vi "Generate Signature.vi"(8 "error in (no error)":errorcluster, 9 "Key":string, 10 "Message":string, 11 "HMAC in":refnum<class "HMAC.lvclass">) -> (0 "error out":errorcluster, 2 "Signature":string, 3 "HMAC out":refnum<class "HMAC.lvclass">)   [LabVIEW 2018, in "Crypto.lvlib" / "HMAC.lvclass"]
uses:
  HMAC.lvclass
  HMAC.lvclass/HMAC.ctl
  Hash/Hash.lvclass
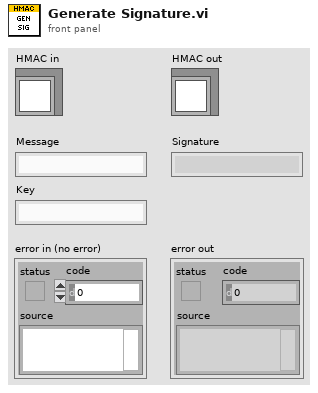
[diagram p1: front panel]
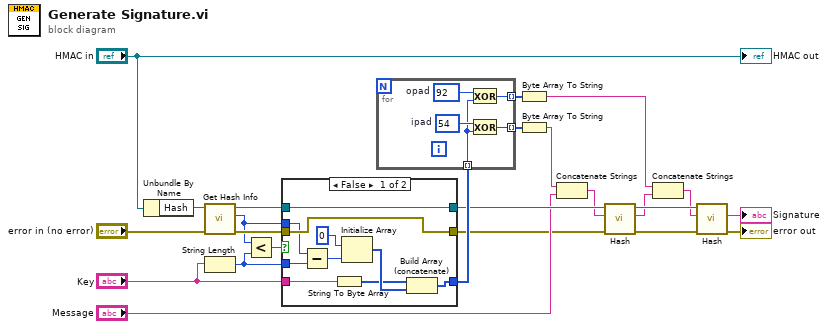
[diagram p0: block diagram]
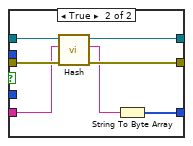
[diagram p2: hidden frame]
diagram:
  n1 = Unbundle By Name("HMAC in") -> ("Hash"=w1:refnum<class "Hash.lvclass">)
  n2 = call-dynamic "Get Hash Info.vi"("error in (no error)"="error in (no error)", "Hash in"=w1) -> ("error out"=w7:errorcluster, "Blocksize (Bytes)"=w3:i32, "Hash out"=w24:refnum<class "Hash.lvclass">)  [unwired: 6 in, 1 out]
  n3 = String Length(string="Key") -> (length=w22:i32)
  n4 = Less?(x=w3, y=w22) -> (x < y?=w23:bool)
  n5 = case shown="False" w23 {
    tunnel: w24 -> [w30 w41]
    tunnel: w22 -> [w33 _]
    tunnel: [w30 w40] -> w17
    tunnel: [w26 w39] -> w20
    tunnel: "Key" -> [w28 w35]
    tunnel: w3 -> [w25 _]
    tunnel: w7 -> [w34 w38]
    tunnel: [w34 w37] -> w6
    frame False {
      n6 = Subtract(x=w25, y=w33) -> (x-y=w32:i32)
      n7 = String To Byte Array(string=w28) -> (unsigned byte array=w27:u8[])
      n8 = Initialize Array(u8 0, w32) -> (w29:u8[])
      n9 = Build Array (concatenate)(w27, w29) -> (w26:u8[])
    }
    frame True {
      n10 = call-dynamic "Hash.vi"("error in (no error)"=w38, "Message"=w35, "Hash in"=w41) -> ("error out"=w37:errorcluster, "Hash"=w36:string, "Hash out"=w40:refnum<class "Hash.lvclass">)  [unwired: 6 in]
      n11 = String To Byte Array(string=w36) -> (unsigned byte array=w39:u8[])
    }
  }
  n12 = for {
    tunnel: w20 -> [w44] mode=indexing
    tunnel: [w43] -> w19 mode=indexing
    tunnel: [w42] -> w18 mode=indexing
    w45 = u8 92  # opad
    w46 = u8 54  # ipad
    n13 = Exclusive Or(1:w44, 2:w45) -> (0:w43:u8)
    n14 = Exclusive Or(1:w44, 2:w46) -> (0:w42:u8)
  }
  n15 = Byte Array To String(unsigned byte array=w19) -> (string=w13:string)
  n16 = Byte Array To String(unsigned byte array=w18) -> (string=w15:string)
  n17 = Concatenate Strings(w15, "Message") -> (w14:string)
  n18 = call-dynamic "Hash.vi"("error in (no error)"=w6, "Message"=w14, "Hash in"=w17) -> ("error out"=w9:errorcluster, "Hash"=w10:string, "Hash out"=w12:refnum<class "Hash.lvclass">)  [unwired: 6 in]
  n19 = Concatenate Strings(w13, w10) -> (w11:string)
  n20 = call-dynamic "Hash.vi"("error in (no error)"=w9, "Message"=w11, "Hash in"=w12) -> ("error out"=→"error out":errorcluster, "Hash"=→"Signature":string)  [unwired: 6 in, 1 out]
  "HMAC out" <- "HMAC in"
